vi "Write Data.vi"   [LabVIEW 2019, in "D2XX-lv.lvlib"]
doc: "Write data to the open device."
uses:
  D2XX-lv.lvlib
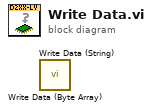
[diagram p0: block diagram]
diagram:
  n1 = call "Write Data (Byte Array).vi"() -> ()  [unwired: 9 in, 3 out]
  n2 = call "Write Data (String).vi"() -> ()  [unwired: 9 in, 3 out]
